vi "NI6071E.StartDAQ.vi"(0 "i ref in":refnum<vi>, 1 "Use attribute data (f)":bool, 2 "PPMA DAQ Start":T3={"scan rate (40000 scans/sec)"=1.0, "trigger type (analog)"=enum."no trigger", "edge or slope \n(rising)"=enum."falling", "number of buffers to acquire (1)"=1, "analog chan (PFI0) & level (2.00)"={"trigger channel (empty)"="", "level (0.0)"=0.0}, "[additional trig params]"={"hysteresis (0.0)"=-1.0, "coupling (no change:0)"=enum."no change", "delay (0 sec)"=0.0, "skip count (0)"=0, "time limit (0 sec)"=0.0}} {"[additional trig params]"."time limit (0 sec)" format="%0.2f"; "[additional trig params]"."delay (0 sec)" format="%0.2f"; "[additional trig params]"."hysteresis (0.0)" format="%0.2f"; "analog chan (PFI0) & level (2.00)"."level (0.0)" format="%0.2f"; "scan rate (40000 scans/sec)" format="%0.2f"}, 4 "timeout ms (60000)":i32=60000, 5 "error in (no error)":errorcluster) -> (14 "i ref out":refnum<vi>, 19 "error out":errorcluster)   [LabVIEW 2014, in "NI6071E.lvlib"]
uses:
  NI6071E.lvlib
  NI6071EStart.ctl
  NI6071ECommandCluster.ctl
  NI6071ECommand.ctl
panel:
  in  "PPMA Command":T1=enum."ConfigureDAQ"
  in  "PPMA Command Cluster":T2
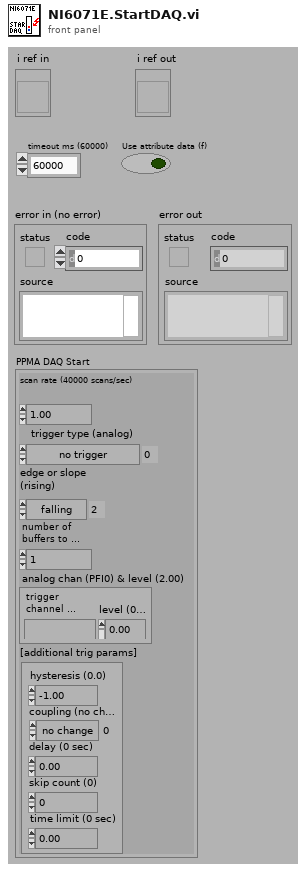
[diagram p1: front panel]
types:
  T1 = typedef "NI6071E.lvlib/NI6071ECommand.ctl" = enum16{"Ping", "Reset", "ConfigureDAQ", "StartDAQ", "StopDAQ", "GetDAQStatus", "ReadData", "SaveData", "CloseConnection"}
  T2 = typedef "NI6071E.lvlib/NI6071ECommandCluster.ctl" = cluster{"Command":string, "Data":string, "error out":errorcluster}
  T3 = typedef "NI6071E.lvlib/NI6071EStart.ctl" = cluster{"scan rate (40000 scans/sec)":sgl, "trigger type (analog)":enum16{"no trigger", "analog", "digital A", "digital A & B", "scan clock gate"}, "edge or slope \n(rising)":enum16{"no change", "rising", "falling"}, "number of buffers to acquire (1)":i32, "analog chan (PFI0) & level (2.00)":cluster{"trigger channel (empty)":string, "level (0.0)":sgl}, "[additional trig params]":cluster{"hysteresis (0.0)":sgl, "coupling (no change:0)":enum16{"no change", "DC", "AC"}, "delay (0 sec)":sgl, "skip count (0)":i32, "time limit (0 sec)":sgl}}
  T4 = typedef "NI6071E.lvlib/NI6071E.i attribute.ctl" = cluster{"NI6071E Server":string, "Port":u16, "NI6071E Config":T5, "NI6071E Start":T3, "Waveforms":waveform(dbl)[], "RT Error":errorcluster, "NI6071E Read":T6, "connection ID":refnum<k5>, "DAQ Status":string, "device (1)":i16, "DAQ Status Service ID":i32}
  T5 = typedef "NI6071E.lvlib/NI6071EConfig.ctl" = cluster{"device (1)":i16, "channels (0)":tag[], "buffer size (1000 scans)":i32, "[number of buffers] (1)":i32, "measurement mode structure":cluster{"measurement mode":u16, "reserved":u32}, "input limits (no change)":cluster{"high limit (0.0)":sgl, "low limit (0.0)":sgl}[], "coupling & input config (no change:0)":cluster{"coupling (no change:0)":enum16{"no change", "DC", "AC", "GND", "internal ref."}, "input config (no change:0)":u16}[]}
  T6 = typedef "NI6071E.lvlib/NI6071ERead.ctl" = cluster{"time limit in sec (-1:auto calculate)":sgl, "number of scans to read (-1:all)":i32}
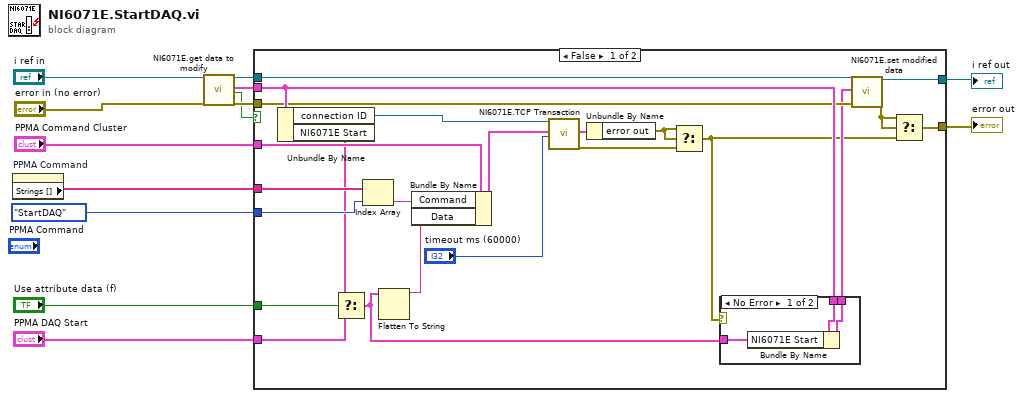
[diagram p0: block diagram]
diagram:
  n1 = property on="PPMA Command" class="Enum (strict)"() -> ("Strings []"=w5:string[])  [unwired: 2 in, 2 out]
  n2 = call "NI6071E.get data to modify.vi"("i ref in"="i ref in", "error in (no error)"="error in (no error)") -> ("i ref out"=w9:refnum<vi>, "i attribute"=w11:T4, "timed out"=w1:bool, "error out"=w10:errorcluster)  [unwired: 14 in]
  n3 = case shown="False" w1 {
    tunnel: w11 -> [w36 _]
    tunnel: w10 -> [w35 w41]
    tunnel: w9 -> [w34 w42]
    tunnel: [w33 w42] -> w8
    tunnel: [w31 w41] -> w7
    tunnel: "PPMA Command Cluster" -> [w28 _]
    tunnel: w5 -> [w26 _]
    tunnel: NI6071ECommand."StartDAQ" ("PPMA Command") -> [w25 _]
    tunnel: "PPMA DAQ Start" -> [w17 _]
    tunnel: "Use attribute data (f)" -> [w14 _]
    frame False {
      n4 = Unbundle By Name(w36) -> ("connection ID"=w29:refnum<k5>, "NI6071E Start"=w15:T3)
      n5 = Select(t=w15, s=w14, f=w17) -> (s? t:f=w16:T3)
      n6 = Index Array(array=w26, index=w25) -> (element=w24:string)
      n7 = Flatten To String(anything=w16) -> (data string=w23:string)  [unwired: 3 in, 2 out]
      n8 = Bundle By Name(cluster=w28, "Command"=w24, "Data"=w23) -> (w27:T2)
      n9 = call "NI6071E.TCP Transaction.vi"("connection ID in"=w29, "NI6071E Command Cluster"=w27, "timeout ms (25000)"="timeout ms (60000)") -> ("NI6071E Response"=w21:T2, "error out"=w19:errorcluster)  [unwired: 14 in, 1 out]
      n10 = Unbundle By Name(w21) -> ("error out"=w20:errorcluster)
      n11 = Select(t=w20, s=w20, f=w19) -> (s? t:f=w18:errorcluster)
      n12 = case shown="No Error" w18 {
        tunnel: w36 -> [w39 w40]
        tunnel: [w38 w40] -> w30
        tunnel: w16 -> [w37 _]
        frame No Error {
          n13 = Bundle By Name(cluster=w39, "NI6071E Start"=w37) -> (w38:T4)
        }
        frame Error {
        }
      }
      n14 = call "NI6071E.set modified data.vi"("i ref in"=w34, "i attribute"=w30, "error in (no error)"=w35) -> ("i ref out"=w33:refnum<vi>, "error out"=w32:errorcluster)  [unwired: 15 in]
      n15 = Select(t=w32, s=w32, f=w18) -> (s? t:f=w31:errorcluster)
    }
    frame True {
    }
  }
  "i ref out" <- w8
  "error out" <- w7
